vi "Network control test 2 reader.vi"() -> ()   [LabVIEW 2018]
uses:
  <vilib>/dex/Stream Element Allocation Mode.ctl
panel:
  in  "writer url":string="//192.168.0.57/"
  in  "Stop Button":bool
  out "number (0 to 1)":dbl
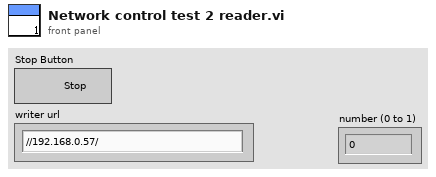
[diagram p1: front panel]
types:
  T1 = typedef "Stream Element Allocation Mode.ctl" = u32
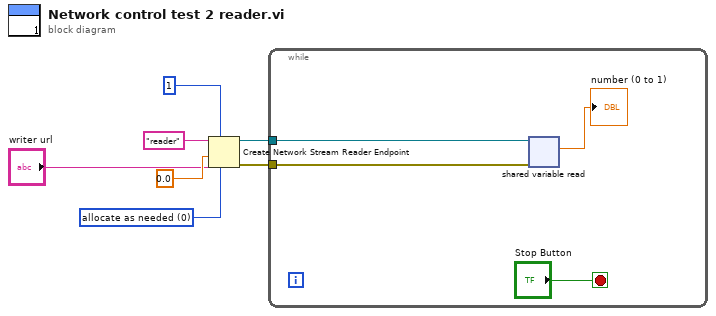
[diagram p0: block diagram]
diagram:
  w6 = T1 0 items=["allocate as needed", "pre-allocate"] ("element allocation mode")
  n1 = Create Network Stream Reader Endpoint(6:w6, 7:1 ("writer buffer size"), 9:0.0, 10:"writer url", 11:"reader" ("writer name")) -> (0:w3:errorcluster, 3:w4:refnum<k21>)  [unwired: 2 in]
  n2 = while {
    tunnel: w4 -> [w8]
    tunnel: w3 -> [w10]
    stop <- "Stop Button" stop-if-true
    n3 = shared-variable-read(w8, w10) -> (→"number (0 to 1)":dbl)  [unwired: 1 in, 3 out]
  }
